vi "Transmit EMS Message.vi"(8 "error in (no error)":errorcluster, 10 "Message":T1, 11 "SCADA Communications in":refnum<class "SCADA Communications.lvclass">) -> (0 "error out":errorcluster, 3 "SCADA Communications out":refnum<class "SCADA Communications.lvclass">)   [LabVIEW 2015, in "SCADA Communcations Actor.lvlib" / "SCADA Communications.lvclass"]
uses:
  SCADA Communications.lvclass
  Controls/EMS Message Cluster.ctl
  TCPIP Communications Framework/TCPIP Communications/TCPIP Communications.lvclass
  Utilities/Message Strings.llb/Message String Utilities.lvlib
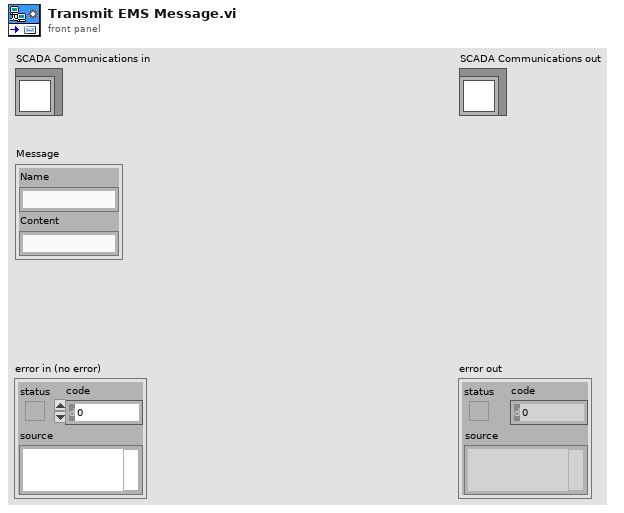
[diagram p1: front panel]
types:
  T1 = typedef "SCADA Communcations Actor.lvlib/SCADA Communications.lvclass/EMS Message Cluster.ctl" = cluster{"Name":string, "Content":string}
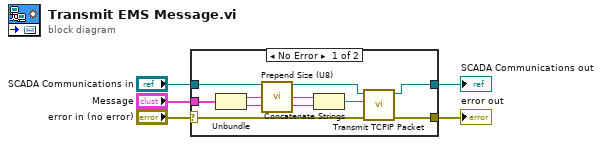
[diagram p0: block diagram]
diagram:
  n1 = case shown="No Error" "error in (no error)" {
    selector: "error in (no error)" -> [w12 w16]
    tunnel: [w11 w16] -> w4
    tunnel: [w13 w15] -> w2
    tunnel: "SCADA Communications in" -> [w14 w15]
    tunnel: "Message" -> [w10 _]
    frame No Error {
      n2 = Unbundle(w10) -> ("Name"=w7:string, "Content"=w9:string)
      n3 = call "Prepend Size (U8).vi"("String in"=w7) -> ("String out"=w6:string)
      n4 = Concatenate Strings(w6, w9) -> (w8:string)
      n5 = call "Transmit TCPIP Packet.vi"("error in (no error)"=w12, "Packet"=w8, "TCPIP Communications in"=w14) -> ("error out"=w11:errorcluster, "TCPIP Communications out"=w13:refnum<class "SCADA Communications.lvclass">)  [unwired: 7 in]
    }
    frame Error {
    }
  }
  "error out" <- w4
  "SCADA Communications out" <- w2
